vi "get All Data.vi"(0 "identifier":string, 1 "data_number":u32, 2 "id":u32[](array[numeric]), 3 "values":u16[](array[numeric]), 4 "error in (no error)":errorcluster, 5 "spectra_size":u32, 6 "Board":u16, 7 "stats":dbl[](array[numeric]), 9 "advstats":u64[](array[numeric])) -> (11 "advstats out":u64[](array[numeric]), 13 "stats out":dbl[](array[numeric]), 14 "function return":bool, 15 "data_number out":u32, 16 "id out":u32[](array[numeric]), 17 "values out":u16[](array[numeric]), 18 "error out":errorcluster, 19 "spectra_size out":u32)   [LabVIEW 2015, in "XGL_DPP.lvlib"]
doc: "EXTERN DECLSPEC bool CALL_CONV getAllData(const char* identifier,\n unsigned short Board,\n unsigned short int* values,\n unsigned long int* id,\n double* stats,\n unsigned long long int* advstats,\n unsigned int& spectra_size,\n unsigned int& data_number\n);"
uses:
  XGL_DPP.lvlib
  XGL_DPP.dll
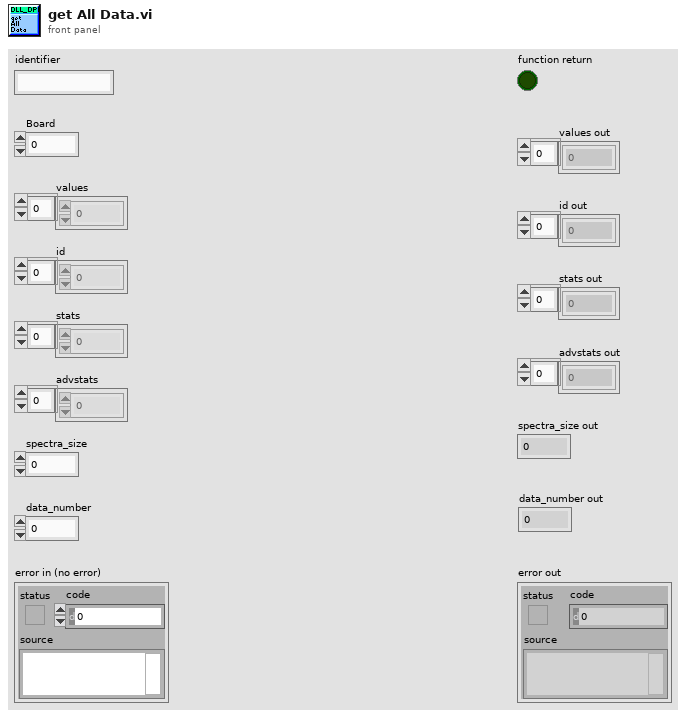
[diagram p1: front panel]
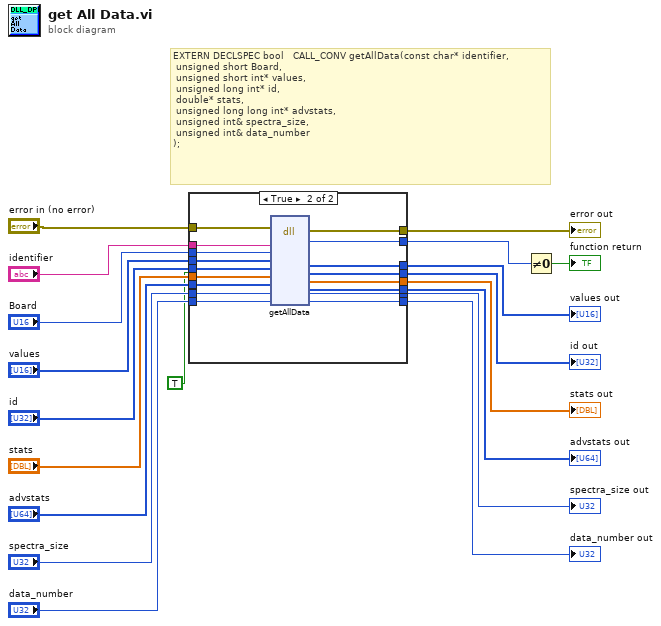
[diagram p0: block diagram]
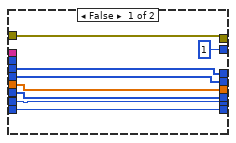
[diagram p2: hidden frame]
diagram:
  # "EXTERN DECLSPEC bool   CALL_CONV getAllData(const char* identifier,\n unsigned short Board,\n unsigned short int* values,\n unsigned long int* id,\n double* stats,\n unsigned long long int* advstats,\n unsigned int& spectra_size,\n unsigned int& data_number\n);"
  n1 = case shown="True" TRUE {
    tunnel: [u8 1 ("return type") w44] -> w18
    tunnel: "identifier" -> [_ w43]
    tunnel: "Board" -> [_ w42]
    tunnel: "spectra_size" -> [w21 w41]
    tunnel: [w21 w40] -> w14
    tunnel: "data_number" -> [w20 w39]
    tunnel: [w20 w38] -> w12
    tunnel: "error in (no error)" -> [w27 w37]
    tunnel: [w27 w36] -> w10
    tunnel: "values" -> [w25 w35]
    tunnel: [w22 w34] -> w8
    tunnel: [w25 w33] -> w7
    tunnel: [w23 w32] -> w6
    tunnel: "id" -> [w23 w31]
    tunnel: [w24 w30] -> w4
    tunnel: "stats" -> [w24 w29]
    tunnel: "advstats" -> [w22 w28]
    frame False {
    }
    frame True {
      n2 = dll-call lib="D:/Users/XRF/Desktop/Dante_acquire4/libs/Dante/XGL_DPP.*" fn="getAllData"(error in=w37, "identifier"=w43, "Board"=w42, "values"=w35, "id"=w31, "stats"=w29, "advstats"=w28, "spectra_size"=w41, "data_number"=w39) -> (error out=w36:errorcluster, "return type"=w44:u8, "values"=w33:u16[], "id"=w32:u32[], "stats"=w30:dbl[], "advstats"=w34:u64[], "spectra_size"=w40:u32, "data_number"=w38:u32)  [unwired: 4 in, 1 out]
    }
  }
  "spectra_size out" <- w14
  "data_number out" <- w12
  "error out" <- w10
  "values out" <- w7
  "id out" <- w6
  "stats out" <- w4
  "advstats out" <- w8
  n3 = Not Equal To 0?(x=w18) -> (x != 0?=→"function return":bool)
